vi "SDG60ConfArbWaveform3.vi"(1 "DDS/TArb 0: DDS":i32(ring) items=["DDS", "TrueArb"], 2 "Interpolation 0: Zero-order":i32(ring) items=["Zero-Order", "Linear", "Sinc", "Sin27", "Sinc13"], 3 "Offset (0.00 V)":dbl min=-10.0 max=10.0 format="%#_15g", 5 "Select Channel (1:Channel 1)":i32(ring)=1 items=["Channel 1"=1, "Channel 2"=2], 7 "Amplitude(0.1 Vpp)":dbl=0.1 min=0.001 max=20.0 step=1.0 format="%#.15f", 9 "Freq/SR/P (1 Hz)":dbl=1.0 min=1e-06 max=160000000.0 step=1.0 format="%#.15g", 12 "Select Freq/SR/P (0:Freq)":i32(ring) items=["Frequency", "Sample Rate", "Period"], 13 "Phase (0 deg)":dbl min=-360.0 max=360.0 format="%#.15g") -> ()   [LabVIEW 2022 SP3]
doc: "Sets the waveform parameters for an arbitrary waveform. This VI should be called after <b>Create Arbitrary Waveform.vi</b> (for user defined arbitrary waveform) and <b>Select Arbitrary Waveform.vi</b>"
uses:
  <vilib>/addons/zeromq/socket_type.ctl
  <vilib>/addons/zeromq/zmq_context.lvclass
  <vilib>/addons/zeromq/zmq_socket.lvclass
  <vilib>/addons/zeromq/zeromq.lvlib
panel:
  out "Python response":string
  # "Must precede with SDG60SelectArbitraryWFM\nMay take time (~20s) if WFM is large"
  # "Sinc type interpolations use virtual keys\nVirtual keys not used for zero-hold & linear\nInterpolation method, is only for TrueArb\nIf still selected, generator will not make any parameter changes"
  # "Range: 2mVpp-20Vpp. \n6 digits precision"
  # "Range: -10V-10V\n6 digits precision"
  # "Freq (DDS): 1uHz-50MHz \nFreq (TrueArb): 1uHz- Max depends on WFM length\nSR: 1uS/s-300MSa/s\nP: 20ns-1Ms\n10 Digit precision for F & SR\n6 Digit precision for P"
  # "May need more testing, as had issues\nwhere some of the parameters didn't go\nthrough the first time round"
  # "For TrueArb use only F or SR \nFor DDS use F or P\nMay take time (seconds to tens of secons!) to switch to TrueArb if WFM is large"
  # "Range -360..360deg, larger values will be warped to this range. Resolution 0.0001 deg"
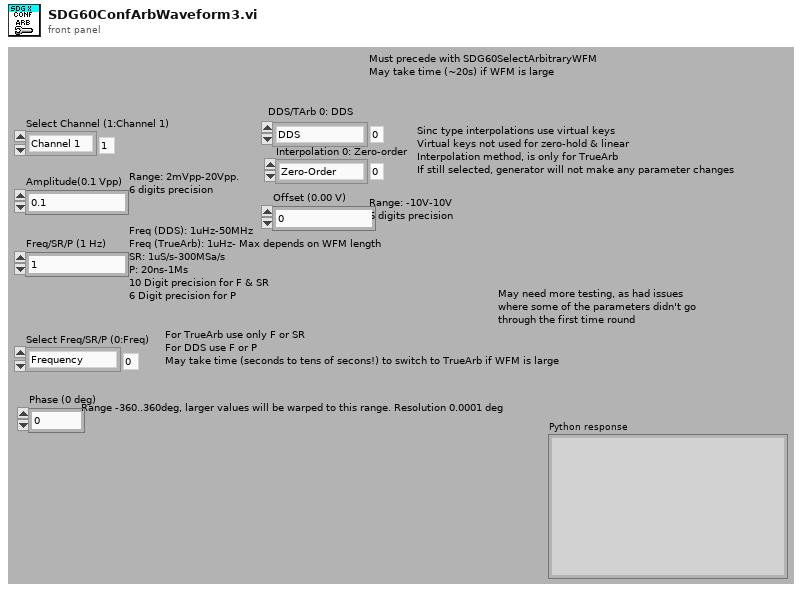
[diagram p1: front panel]
types:
  T1 = typedef "zeromq.lvlib/socket_type.ctl" = enum8{"ZMQ_PAIR", "ZMQ_PUB", "ZMQ_SUB", "ZMQ_REQ", "ZMQ_REP", "ZMQ_DEALER", "ZMQ_ROUTER", "ZMQ_PULL", "ZMQ_PUSH", "ZMQ_XPUB", "ZMQ_XSUB", "ZMQ_STREAM", "ZMQ_SERVER", "ZMQ_CLIENT", "ZMQ_RADIO", "ZMQ_DISH", "ZMQ_GATHER", "ZMQ_SCATTER", "ZMQ_DGRAM"}
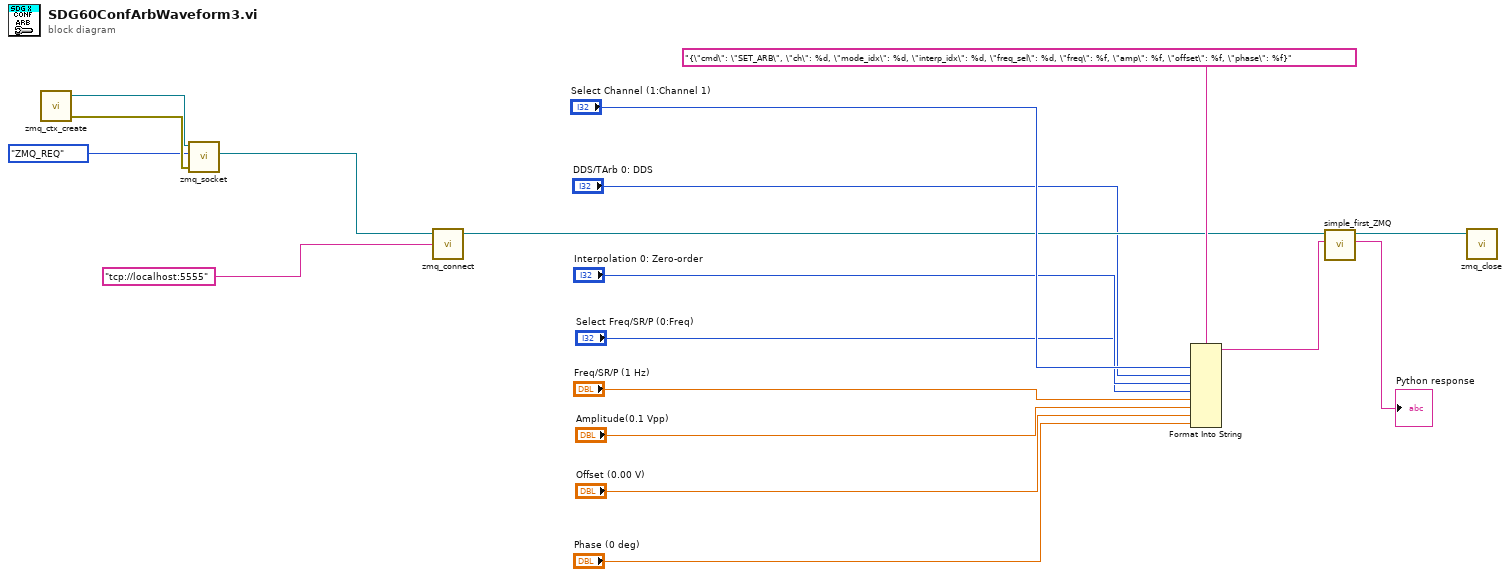
[diagram p0: block diagram]
diagram:
  n1 = call <vilib>:"zmq_ctx_create.vi"() -> ("error out"=w11:errorcluster, "context out"=w12:refnum<class "zmq_context.lvclass">)  [unwired: 4 in]
  n2 = call <vilib>:"zmq_socket.vi"("error in"=w11, "socket type"=socket_type."ZMQ_REQ", "context in"=w12) -> ("socket out"=w8:refnum<class "zmq_socket.lvclass">)  [unwired: 2 in, 2 out]
  n3 = call <vilib>:"zmq_connect.vi"("endpoint"="tcp://localhost:5555", "socket in"=w8) -> ("socket out"=w7:refnum<class "zmq_socket.lvclass">)  [unwired: 2 in, 1 out]
  n4 = Format Into String(format string="{\"cmd\": \"SET_ARB\", \"ch\": %d, \"mode_idx\": %d, \"interp_idx\": %d, \"freq_sel\": %d, \"freq\": %f, \"amp\": %f, \"offset\": %f, \"phase\": %f}", "Select Channel (1:Channel 1)", "DDS/TArb 0: DDS", "Interpolation 0: Zero-order", "Select Freq/SR/P (0:Freq)", "Freq/SR/P (1 Hz)", "Amplitude(0.1 Vpp)", "Offset (0.00 V)", "Phase (0 deg)") -> (resulting string=w6:string)  [unwired: 2 in, 1 out]
  n5 = call "simple_first_ZMQ.vi"("Raw command"=w6, "ZMQ socket in"=w7) -> ("Python response"=→"Python response":string, "ZMQ socket out"=w4:refnum<class "zmq_socket.lvclass">)  [unwired: 4 in]
  n6 = call <vilib>:"zmq_close.vi"("socket"=w4) -> ()  [unwired: 4 in, 1 out]
